vi "Image_Save_Dequeue.vi"(0 "Data":T2={"system"={"info"={"menuSelect"=0, "version"=0, "serial"="Test Sample", "captureActive"=FALSE, "captureBegin"=FALSE, "emptyAndRefill"=FALSE}, "userInfo"={"operatorName"="", "date"=timestamp(2713993200 s since 1904-01-01)}, "camera"={"exposureTime"=0, "aperture"=enum."Item 0", "framerate"=0, "framerateMax"=500, "legacyAttributes"=FALSE}}, "connections"={"arduino"={"connection"="MRJ", "status"=FALSE, "openState"=FALSE, "emptyStart"=0}, "pump"={"connection"="MRJ", "status"=FALSE, "command"="", "dispenseSpeed"=100, "flushSize"=100}, "camera"={"cam1"={"connection"="", "status"=FALSE}, "cam2"={"connection"="", "status"=FALSE}}}, "queue"={"process"={"cam1"=refnum, "cam2"=refnum, "queueSize"=0}, "save"={"cam1"=refnum, "cam2"=refnum, "queueSize"=0}, "overloadThreshold"=0}, "imageProcess"={"cam1"={"preAllocation"={"image"="Station", "originalDisplay"="Station", "originalRgb"="Station", "binary"="Station", "save"="Station", "calibrationFull"=refnum, "calibrationDetect"=refnum}, "calibration"={"pathFull"=path "C:/Users/au540322/Desktop/IHS_Project/images/Debris/Debris_0/Debris_0_2019_06_01-23-32-49-686.PNG", "pathDetect"=path "C:/Users/au540322/Desktop/IHS_Project/images/Debris/Debris_0/Debris_0_2019_06_01-23-32-49-686.PNG", "ROI"={"Left"=0, "Top"=0, "Right"=0, "Bottom"=0, "Rotation"=0.0}}}, "cam2"={"preAllocation"={"image"=refnum, "originalDisplay"=refnum, "originalRgb"=refnum, "binary"=refnum, "save"=refnum, "calibrationFull"=refnum, "calibrationDetect"=refnum}, "calibration"={"pathFull"=path "C:/Users/au540322/Desktop/IHS_Project/images/Debris/Debris_0/Debris_0_2019_06_01-23-32-49-686.PNG", "pathDetect"=path "C:/Users/au540322/Desktop/IHS_Project/images/Debris/Debris_0/Debris_0_2019_06_01-23-32-49-686.PNG", "ROI"={"Left"=0, "Top"=0, "Right"=0, "Bottom"=0, "Rotation"=0.0}}}, "process"={"planeExtract"=refnum, "planeSubtract"=refnum, "cropMask"=refnum}, "detection"={"sampleTimeout"=500, "sizeThreshold"=500, "detectionRegionPct"=0.0}}, "sampleData"={"sampleId"="", "projectId"="", "voucherID"="", "speciesName"="", "collectionDate"=timestamp(2713993200 s since 1904-01-01), "sampleStation"="", "location"="", "lat"=0.0, "lon"=0.0, "determiner"="", "sex"="", "otherNotes"=""}, "Session In"=""} {"sampleData"."collectionDate" format="%<%Y-%m-%d>T"; "imageProcess"."detection"."sizeThreshold" min=1; "imageProcess"."cam2"."calibration"."ROI"."Rotation" format="%.2f"; "imageProcess"."cam2"."calibration"."ROI"."Left" scale=0.0..1024.0; "imageProcess"."cam2"."calibration"."ROI"."Right" scale=0.0..1024.0; "imageProcess"."cam1"."calibration"."ROI"."Rotation" format="%.2f"; "imageProcess"."cam1"."calibration"."ROI"."Left" scale=0.0..1024.0; "imageProcess"."cam1"."calibration"."ROI"."Right" scale=0.0..1024.0; "queue"."overloadThreshold" min=1; "queue"."save"."queueSize" min=1; "queue"."process"."queueSize" min=1; "connections"."pump"."flushSize" min=1; "connections"."pump"."dispenseSpeed" min=1; "system"."camera"."framerateMax" min=1; "system"."userInfo"."date" format="%<%Y-%m-%dT%H:%M:%S+%z>T"; "system"."info"."version" items=["Standard", "XL"]; "system"."info"."menuSelect" items=["Session Data", "Extended Setup", "Buffer", "Camera", "Dispenser", "Stats", "Connections"]}, 2 "Camera":T5, 3 "Old":i32, 4 "cam1_prev":u32, 5 "Other":i32, 6 "Queue active":bool, 7 "cam2_prev":u32) -> (16 "timed out?":bool, 17 "Sample Data":dbl[](array[numeric]), 20 "# elements in queue":i32, 22 "State out":i32, 23 "Image Save 1":T1, 24 "cam1_count":u32, 25 "Image Save 2":T1, 26 "Last image":bool, 27 "cam2_count":u32)   [LabVIEW 2022 SP3]
uses:
  Camera_ID.ctl
  controls/Data.ctl
  <vilib>/userdefined/High Color/IMAQdx.ctl
  <vilib>/vision/Image Controls.llb/IMAQ Image.ctl
panel:
  out "error out":errorcluster
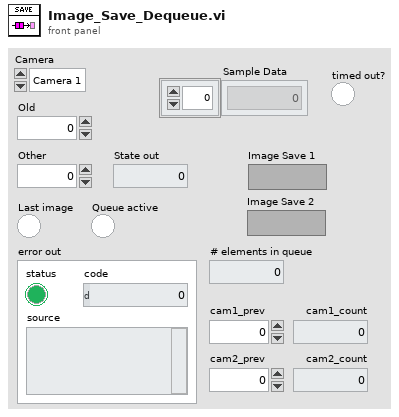
[diagram p1: front panel]
types:
  T1 = typedef "IMAQ Image.ctl" = refnum<image>
  T2 = typedef "Data.ctl" = cluster{"system":cluster{"info":cluster{"menuSelect":u16, "version":u16, "serial":string, "captureActive":bool, "captureBegin":bool, "emptyAndRefill":bool}, "userInfo":cluster{"operatorName":string, "date":timestamp}, "camera":cluster{"exposureTime":i32, "aperture":enum32{"Item 0", "Item 1", "Item 2", "Item 3"}, "framerate":i32, "framerateMax":i32, "legacyAttributes":bool}}, "connections":cluster{"arduino":cluster{"connection":refnum<visa-resource-name>, "status":bool, "openState":bool, "emptyStart":u32}, "pump":cluster{"connection":refnum<visa-resource-name>, "status":bool, "command":string, "dispenseSpeed":i32, "flushSize":i32}, "camera":cluster{"cam1":cluster{"connection":T3, "status":bool}, "cam2":cluster{"connection":T3, "status":bool}}}, "queue":cluster{"process":cluster{"cam1":refnum<queue>, "cam2":refnum<queue>, "queueSize":i32}, "save":cluster{"cam1":refnum<queue>, "cam2":refnum<queue>, "queueSize":i32}, "overloadThreshold":i32}, "imageProcess":cluster{"cam1":cluster{"preAllocation":cluster{"image":T1, "originalDisplay":T1, "originalRgb":T1, "binary":T1, "save":T1, "calibrationFull":T1, "calibrationDetect":T1}, "calibration":cluster{"pathFull":path, "pathDetect":path, "ROI":T4}}, "cam2":cluster{"preAllocation":cluster{"image":T1, "originalDisplay":T1, "originalRgb":T1, "binary":T1, "save":T1, "calibrationFull":T1, "calibrationDetect":T1}, "calibration":cluster{"pathFull":path, "pathDetect":path, "ROI":T4}}, "process":cluster{"planeExtract":T1, "planeSubtract":T1, "cropMask":T1}, "detection":cluster{"sampleTimeout":i32, "sizeThreshold":i32, "detectionRegionPct":dbl}}, "sampleData":cluster{"sampleId":string, "projectId":string, "voucherID":string, "speciesName":string, "collectionDate":timestamp, "sampleStation":string, "location":string, "lat":dbl, "lon":dbl, "determiner":string, "sex":string, "otherNotes":string}, "Session In":T3}
  T3 = typedef "IMAQdx.ctl" = refnum<k21>
  T4 = typedef "IMAQ Rectangle" = cluster{"Left":i32, "Top":i32, "Right":i32, "Bottom":i32, "Rotation":dbl}
  T5 = typedef "Camera_ID.ctl" = enum16{"Camera 1", "Camera 2"}
  T6 = cluster{"Timestamp":string, "Image Pixels (U32)":u32[][], "Prev. sample":i32, "Sample Data":dbl[], "output cluster":cluster{"Global Rectangle":i32[], "Contours":cluster{"ID":enum32{"External", "Internal"}, "Type":u32, "Coordinates":i32[]}[]}}
  T7 = cluster{"Global Rectangle":i32[], "Contours":cluster{"ID":enum32{"External", "Internal"}, "Type":u32, "Coordinates":i32[]}[]}
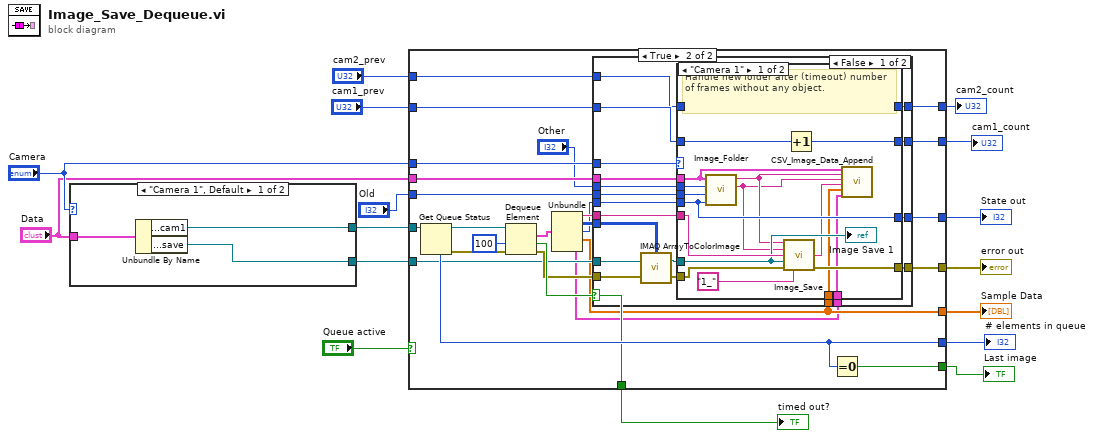
[diagram p0: block diagram]
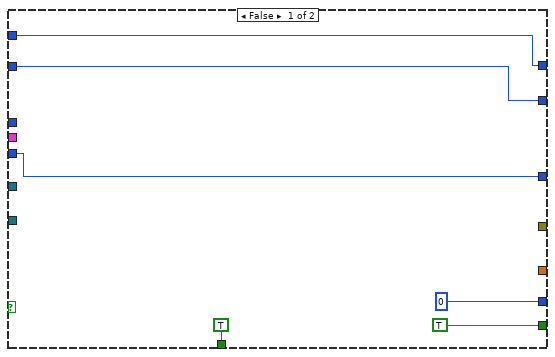
[diagram p2: hidden frame]
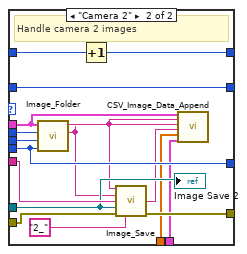
[diagram p3: hidden frame]
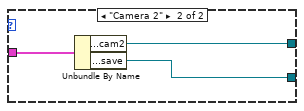
[diagram p5: hidden frame]
diagram:
  n1 = case shown="\"Camera 1\", Default" "Camera" {
    tunnel: [w18 w22] -> w15
    tunnel: "Data" -> [w19 w21]
    tunnel: [w17 w20] -> w5
    frame "Camera 1", Default {
      n2 = Unbundle By Name(w19) -> ("queue.save.cam1"=w18:refnum<queue>, "imageProcess.cam1.preAllocation.save"=w17:T1)
    }
    frame "Camera 2" {
      n3 = Unbundle By Name(w21) -> ("queue.save.cam2"=w22:refnum<queue>, "imageProcess.cam2.preAllocation.save"=w20:T1)
    }
  }
  n4 = case shown="True" "Queue active" {
    tunnel: "Camera" -> [_ w53]
    tunnel: w15 -> [_ w49]
    tunnel: "Data" -> [_ w48]
    tunnel: [0 ("# elements in queue") w47] -> w12
    tunnel: [TRUE w46] -> w11
    tunnel: [_ w45] -> w10
    tunnel: [w26 w40] -> w9
    tunnel: "Old" -> [w26 w39]
    tunnel: [_ w34] -> w7
    tunnel: [TRUE ("timed out?") w37] -> w6
    tunnel: w5 -> [_ w35]
    tunnel: [w24 w32] -> w4
    tunnel: "cam1_prev" -> [w24 w31]
    tunnel: "cam2_prev" -> [w23 w30]
    tunnel: [w23 w29] -> w1
    frame False {
    }
    frame True {
      n5 = Get Queue Status(queue=w49) -> (queue out=w50:refnum<queue>, error out=w43:errorcluster, # elements in queue=w47:i32)  [unwired: 2 in, 5 out]
      n6 = Dequeue Element(queue=w50, timeout in ms (-1)=100, error in (no error)=w43) -> (element=w52:T6, timed out?=w37:bool, error out=w36:errorcluster)  [unwired: 1 out]
      n7 = Unbundle(w52) -> ("Timestamp"=w44:string, "Image Pixels (U32)"=w51:u32[][], "Prev. sample"=w42:i32, "Sample Data"=w34:dbl[], "output cluster"=w33:T7)
      n8 = case shown="False" w37 {
        tunnel: w53 -> [w72 _]
        tunnel: w51 -> [w60 _]
        tunnel: w48 -> [w71 _]
        tunnel: [w70 w109] -> w45
        tunnel: w44 -> [w69 _]
        tunnel: w42 -> [w68 _]
        tunnel: "Other" -> [w67 _]
        tunnel: [w66 w110] -> w40
        tunnel: w39 -> [w65 w110]
        tunnel: w36 -> [w61 w109]
        tunnel: w35 -> [w64 _]
        tunnel: w34 -> [w59 _]
        tunnel: w33 -> [w58 _]
        tunnel: [w57 w108] -> w32
        tunnel: w31 -> [w56 w108]
        tunnel: w30 -> [w55 w107]
        tunnel: [w54 w107] -> w29
        frame False {
          n9 = call "IMAQ ArrayToColorImage"("Image Pixels (U32)"=w60, "Image"=w64, "error in (no error)"=w61) -> ("Image Out"=w63:T1, "error out"=w62:errorcluster)  [unwired: 2 in]
          n10 = case shown="\"Camera 1\"" w72 {
            tunnel: [w89 w106] -> w70
            tunnel: w63 -> [w82 w99]
            tunnel: w71 -> [w81 w98]
            tunnel: w69 -> [w87 w104]
            tunnel: w62 -> [w86 w103]
            tunnel: w68 -> [w83 w100]
            tunnel: w65 -> [w85 w102]
            tunnel: w67 -> [w84 w101]
            tunnel: [w83 w100] -> w66
            tunnel: w59 -> [w77 w94]
            tunnel: w58 -> [w76 w93]
            tunnel: [w75 w90] -> w57
            tunnel: w56 -> [w74 w90]
            tunnel: w55 -> [w73 w92]
            tunnel: [w73 w91] -> w54
            frame "Camera 1" {
              # "Handle new folder after (timeout) number of frames without any object."
              n11 = call "Image_Folder.vi"("New"=w83, "Old"=w85, "Other"=w84, "input cluster"=w81) -> ("Subfolder Name"=w79:string, "Subfolder Path"=w80:string)  [unwired: 6 in]
              n12 = call "Image_Save.vi"("Subfolder path"=w80, "Subfolder Name"=w79, "Timestamp"=w87, "Image in"=w82, "error in"=w86, "Camera"="1_" ("Camera image prefix")) -> ("Image Name"=w78:string, "error out"=w89:errorcluster)  [unwired: 6 in, 2 out]
              n13 = Increment(x=w74) -> (x+1=w75:u32)
              n14 = call "CSV_Image_Data_Append.vi"("input cluster"=w81, "Image path"=w80, "Sample Name"=w79, "Image Name"=w78, "Sample Data"=w77, "ROI Descriptor"=w76) -> ()  [unwired: 14 in]
              "Image Save 1" <- w82
            }
            frame "Camera 2" {
              # "Handle camera 2 images"
              n15 = call "Image_Folder.vi"("New"=w100, "Old"=w102, "Other"=w101, "input cluster"=w98) -> ("Subfolder Name"=w96:string, "Subfolder Path"=w97:string)  [unwired: 6 in]
              n16 = Increment(x=w92) -> (x+1=w91:u32)
              n17 = call "Image_Save.vi"("Subfolder path"=w97, "Subfolder Name"=w96, "Timestamp"=w104, "Image in"=w99, "error in"=w103, "Camera"="2_" ("Camera image prefix")) -> ("Image Name"=w95:string, "error out"=w106:errorcluster)  [unwired: 6 in, 2 out]
              n18 = call "CSV_Image_Data_Append.vi"("input cluster"=w98, "Image path"=w97, "Sample Name"=w96, "Image Name"=w95, "Sample Data"=w94, "ROI Descriptor"=w93) -> ()  [unwired: 14 in]
              "Image Save 2" <- w99
            }
          }
        }
        frame True {
        }
      }
      n19 = Equal To 0?(x=w47) -> (x = 0?=w46:bool)
    }
  }
  "# elements in queue" <- w12
  "Last image" <- w11
  "error out" <- w10
  "State out" <- w9
  "Sample Data" <- w7
  "timed out?" <- w6
  "cam1_count" <- w4
  "cam2_count" <- w1
